vi "Destroy to Session.vi"(8 "Error In":errorcluster, 11 "Known Hosts":refnum<class "Known Hosts.lvclass">) -> (0 "Error Out":errorcluster, 3 "Session":refnum<class "Session.lvclass">)   [LabVIEW 2018, in "Toolkit.lvlib" / "Known Hosts.lvclass"]
doc: "Destroys this Known Hosts object and frees the memory allocated within the libssh2lv shared library for the internal linked list. No other VIs within the Known Hosts class should be executed after this VI has completed."
uses:
  Known Hosts.lvclass
  Session/Session.lvclass
  Known Hosts.lvclass/Known Hosts.ctl
  Session/Session.lvclass/Session.ctl
  SSH/SSH.lvclass/SSH.ctl
  Toolkit.lvlib
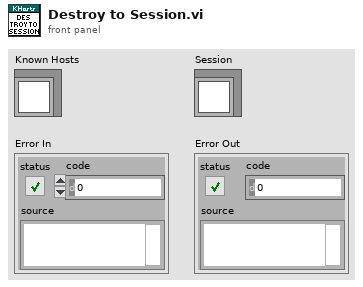
[diagram p1: front panel]
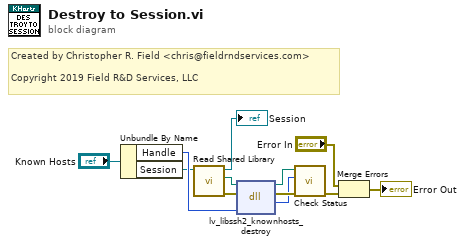
[diagram p0: block diagram]
diagram:
  # "Created by Christopher R. Field <chris@fieldrndservices.com>\n\nCopyright 2019 Field R&D Services, LLC"
  n1 = Unbundle By Name("Known Hosts") -> ("Handle"=w9:u64, "Session"=w4:refnum<class "Session.lvclass">)
  n2 = call "Read Shared Library.vi"("Session In"=w4) -> ("Erorr Out"=w2:errorcluster, "libssh2lv Shared Library"=w3:path, "Session Out"=→"Session":refnum<class "Session.lvclass">)  [unwired: 8 in]
  n3 = dll-call lib="D:/Users/cfield/Code/Field R&D Services/SSH/LV-LIBSSH2/LabVIEW/trunk/src/Toolkit/Support/lv-libssh2.*" fn="lv_libssh2_knownhosts_destroy"(path in=w3, error in=w2, "handle"=w9) -> (path out=w7:path, error out=w8:errorcluster, "status"=w6:i32)  [unwired: 2 in]
  n4 = call "Check Status.vi"("Error In"=w8, "Status"=w6, "libssh2lv Shared Library In"=w7) -> ("Error Out"=w5:errorcluster)  [unwired: 7 in, 1 out]
  n5 = Merge Errors("Error In", w5) -> (→"Error Out":errorcluster)
